vi "GetPowerRvp8.vi"(4 "SpecifyTypeOfDataAcq":string="_", 5 "error in (no error)":errorcluster, 6 "startGate":i32=200 min=1025 step=1, 7 "nGates":i32=500 min=1025 step=1, 8 "nSamples":i32=1000) -> (0 "Comm error":errorcluster, 1 "XML error":errorcluster, 2 "String_of_RVP8_Powers":string, 3 "RVP8_power":T1 {"time" format="%<%H:%M:%S\n%Y/%m/%d>T"})   [LabVIEW 2009]
doc: "Reads the power from the N1911A power meter."
uses:
  Rvp8PowerData.ctl
panel:
  out "XML Response":string="fetch?"
  out "XML commands":string="<TsGrabberCommands>\n  <nSamples>1000</nSamples>\n  <startGate>50</startGate>\n  <nGates>500</nGates>\n  <fastAlternating>true</fastAlternating>\n  <labviewRequest>true</labviewRequest>\n</TsGrabberCommands>\n"
  # "Changed StartGate and nGates to I32 and corrected wiring to each of these (fp:17Aug07).  The defaults must be 1000/500/50 for the calibration programs to work correctly!"
  # "Select ngates and startgate to avoid standard test pulse and Rx switching transient"
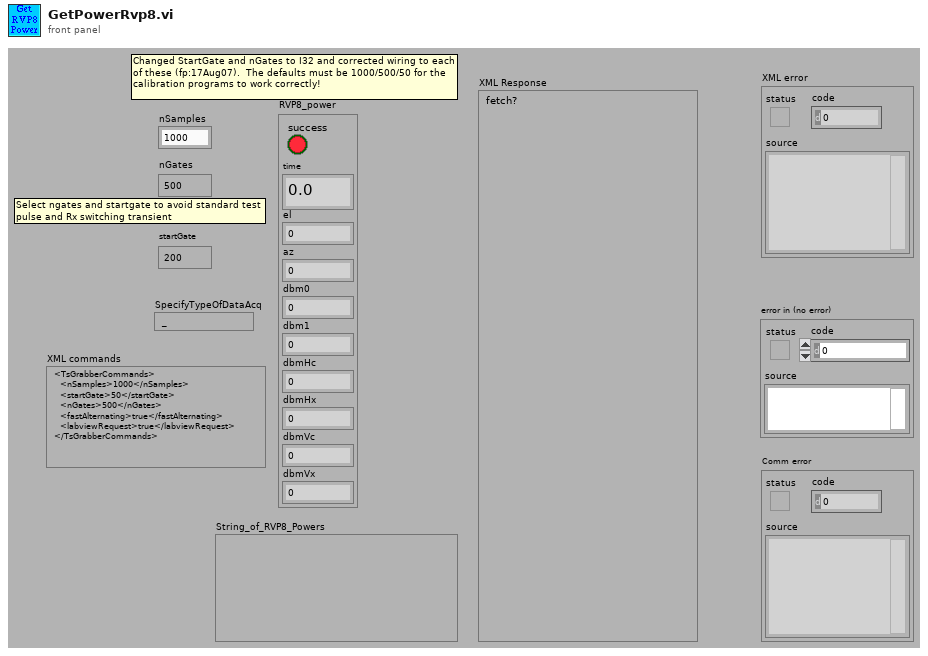
[diagram p1: front panel]
types:
  T1 = typedef "Rvp8PowerData.ctl" = cluster{"success":bool, "time":dbl, "el":dbl, "az":dbl, "dbm0":dbl, "dbm1":dbl, "dbmHc":dbl, "dbmHx":dbl, "dbmVc":dbl, "dbmVx":dbl}
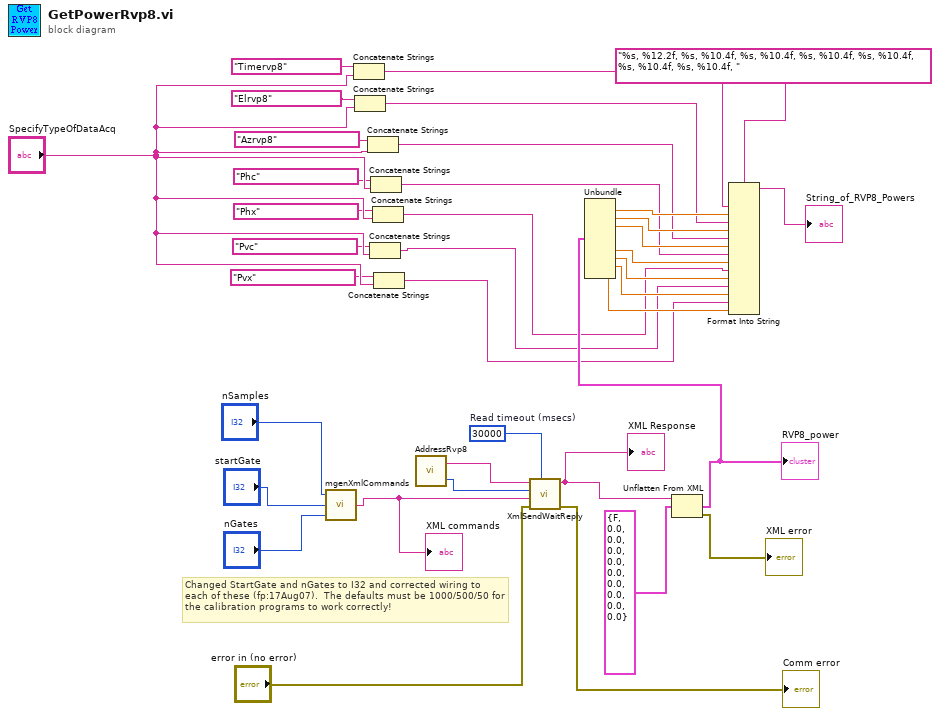
[diagram p0: block diagram]
diagram:
  w34 = 30000  # Read timeout (msecs)
  # "Changed StartGate and nGates to I32 and corrected wiring to each of these (fp:17Aug07).  The defaults must be 1000/500/50 for the calibration programs to work correctly!"
  n1 = call "mgenXmlCommands.vi"("nGates"="nGates", "startGate"="startGate", "nSamples"="nSamples") -> ("TsGrabberCommand"=w29:string)
  "XML commands" <- w29
  n2 = Concatenate Strings("Timervp8", "SpecifyTypeOfDataAcq") -> (w10:string)
  n3 = Concatenate Strings("Elrvp8", "SpecifyTypeOfDataAcq") -> (w9:string)
  n4 = Concatenate Strings("Azrvp8", "SpecifyTypeOfDataAcq") -> (w8:string)
  n5 = Concatenate Strings("Pvc", "SpecifyTypeOfDataAcq") -> (w4:string)
  n6 = Concatenate Strings("Phc", "SpecifyTypeOfDataAcq") -> (w6:string)
  n7 = Concatenate Strings("Phx", "SpecifyTypeOfDataAcq") -> (w5:string)
  n8 = Concatenate Strings("Pvx", "SpecifyTypeOfDataAcq") -> (w3:string)
  n9 = call "AddressRvp8.vi"() -> ("Port"=w36:i32, "IP address"=w35:string)  [unwired: 2 in]
  n10 = call "XmlSendWaitReply.vi"("Read timeout msecs"=w34, "error in (no error)"="error in (no error)", "Command"=w29, "TCP port"=w36, "IP Address"=w35) -> ("Error out"=→"Comm error":errorcluster, "Reply"=w33:string)  [unwired: 4 in]
  "XML Response" <- w33
  n11 = Unflatten From XML(xml string=w33, type=T1 {"success"=FALSE, "time"=0.0, "el"=0.0, "az"=0.0, "dbm0"=0.0, "dbm1"=0.0, "dbmHc"=0.0, "dbmHx"=0.0, "dbmVc"=0.0, "dbmVx"=0.0} ("RVP8_power 2")) -> (value=w24:T1, error out=→"XML error":errorcluster)  [unwired: 1 in]
  "RVP8_power" <- w24
  n12 = Unbundle(w24) -> ("time"=w23:dbl, "el"=w22:dbl, "az"=w7:dbl, "dbmHc"=w21:dbl, "dbmHx"=w20:dbl, "dbmVc"=w19:dbl, "dbmVx"=w18:dbl)  [unwired: 3 out]
  n13 = Format Into String(format string="%s, %12.2f, %s, %10.4f, %s, %10.4f, %s, %10.4f, %s, %10.4f, %s, %10.4f, %s, %10.4f, ", w10, w23, w9, w22, w8, w7, w6, w21, w5, w20, w4, w19, w3, w18) -> (resulting string=→"String_of_RVP8_Powers":string)  [unwired: 2 in, 1 out]
